vi "SSC Digital Calculate Per-Site to Per-Instrument LUT.vi"(0 "Digital SSC In":T2[](array[typedef]), 7 "Sites":i32[](array[numeric])) -> (4 "Per-Site to Per-Instrument LUT":T1[](array[typedef]), 6 "Instrument Count":i32, 8 "Max Sites on Instrument":i32)   [LabVIEW 2019]
uses:
  SSC Digital/SSC Digital.ctl
  Digital 2D Location.ctl
  Shared SubVIs/Trim Whitespace [Inlined].vi
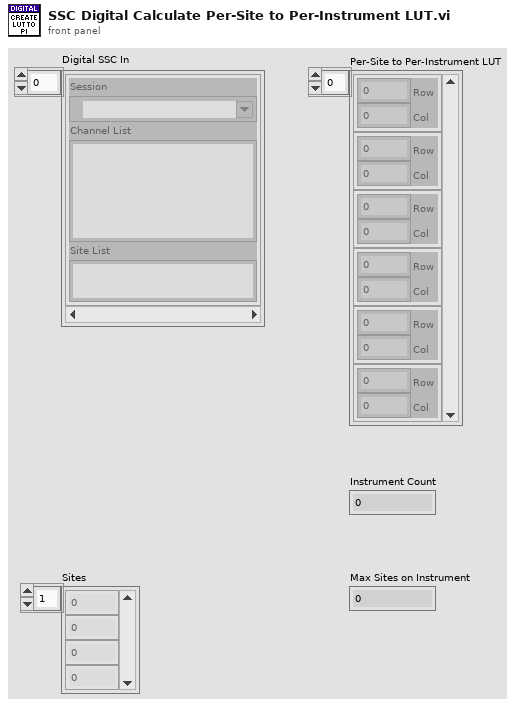
[diagram p1: front panel]
types:
  T1 = typedef "Digital 2D Location.ctl" = cluster{"Row":i32, "Col":i32}
  T2 = typedef "SSC Digital.ctl" = cluster{"Session":refnum<k15>, "Channel List":string, "Site List":string}
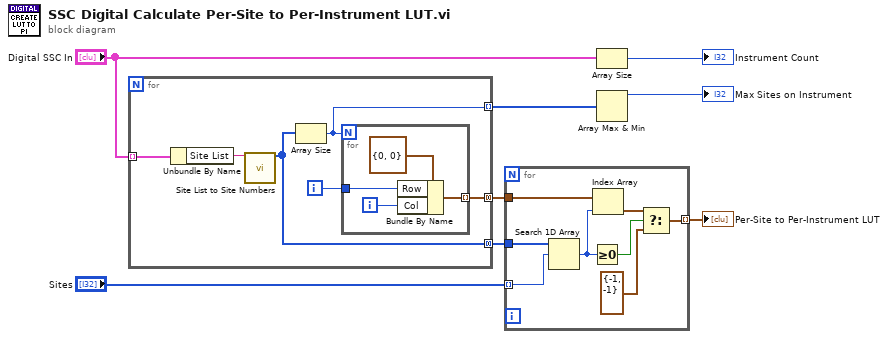
[diagram p0: block diagram]
diagram:
  n1 = for {
    tunnel: "Digital SSC In" -> [w14] mode=indexing
    tunnel: [w10] -> w7 mode=concatenating
    tunnel: [w12] -> w6 mode=concatenating
    tunnel: [w9] -> w2 mode=indexing
    i -> [w13]
    n2 = Unbundle By Name(w14) -> ("Site List"=w11:string)
    n3 = call "Site List to Site Numbers.vi"("Site List"=w11) -> ("Site Numbers"=w10:i32[])  [unwired: 13 in, 1 out]
    n4 = Array Size(array=w10) -> (size(s)=w9:i32)
    n5 = for {
      N: w9 -> [_]
      tunnel: w13 -> [w17]
      tunnel: [w15] -> w12 mode=indexing
      i -> [w16]
      n6 = Bundle By Name(cluster=T1 {"Row"=0, "Col"=0} ("Index"), "Row"=w17, "Col"=w16) -> (w15:T1)
    }
  }
  n7 = for {
    tunnel: "Sites" -> [w26] mode=indexing
    tunnel: [w20] -> w5 mode=indexing
    tunnel: w7 -> [w25]
    tunnel: w6 -> [w24]
    n8 = Search 1D Array(1D array=w25, element=w26) -> (index of element=w23:i32)  [unwired: 1 in]
    n9 = Greater Or Equal To 0?(x=w23) -> (x >= 0?=w22:bool)
    n10 = Index Array(array=w24, index=w23) -> (element=w21:T1)
    n11 = Select(t=w21, s=w22, f=T1 {"Row"=-1, "Col"=-1}) -> (s? t:f=w20:T1)
  }
  "Per-Site to Per-Instrument LUT" <- w5
  n12 = Array Size(array="Digital SSC In") -> (size(s)=→"Instrument Count":i32)
  n13 = Array Max & Min(array=w2) -> (max value=→"Max Sites on Instrument":i32)  [unwired: 3 out]
